vi "enableControls.vi"(8 "Error In":errorcluster, 10 "Disable?":bool, 11 "Controls":refnum<vi>[](array[refnum])) -> (0 "Error Out":errorcluster)   [LabVIEW 2018]
doc: "Sets all the controls in the input array to the \"Enable state\" value."
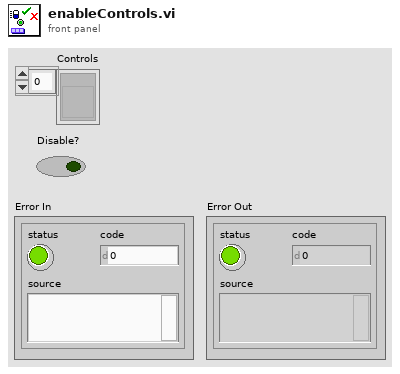
[diagram p1: front panel]
types:
  T1 = enum8{"Enabled", "Disabled", "Disabled and Grayed Out"}
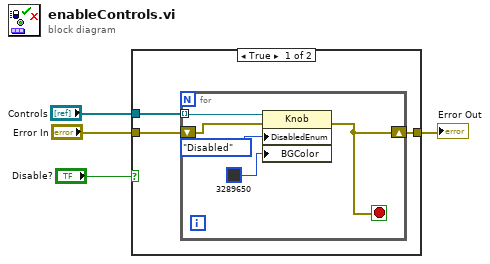
[diagram p0: block diagram]
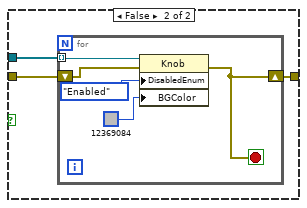
[diagram p2: hidden frame]
diagram:
  n1 = case shown="True" "Disable?" {
    tunnel: "Controls" -> [w7 w15]
    tunnel: [w6 w14] -> w3
    tunnel: "Error In" -> [w5 w13]
    frame True {
      n2 = for {
        tunnel: w7 -> [w12] mode=indexing
        shift-right: [w10] -> w6
        shift-left: w5 -> [w11]
        stop <- w10 stop-if-true
        n3 = property class="Knob"(reference=w12, error in=w11, "DisabledEnum"=T1."Disabled" ("Disabled State"), "BGColor"=u32 3289650) -> (error out=w10:errorcluster)  [unwired: 1 out]
      }
    }
    frame False {
      n4 = for {
        tunnel: w15 -> [w20] mode=indexing
        shift-right: [w18] -> w14
        shift-left: w13 -> [w19]
        stop <- w18 stop-if-true
        n5 = property class="Knob"(reference=w20, error in=w19, "DisabledEnum"=T1."Enabled" ("Disabled State"), "BGColor"=u32 12369084) -> (error out=w18:errorcluster)  [unwired: 1 out]
      }
    }
  }
  "Error Out" <- w3
